vi "PWRMeasureCurrent.vi"(0 "PWR In":refnum<visa-resource-name>, 2 "Channel":string="1", 5 "error in (no error)":errorcluster {"code" format="%.0x"}, 6 "PWRID":u8) -> (14 "PWR Out":refnum<visa-resource-name>, 16 "Current Level (A)":dbl, 19 "error out":errorcluster)   [LabVIEW 2015]
uses:
  <instrlib>/Agilent N6700 Series/Agilent N6700 Series.lvlib
  <instrlib>/Agilent N87XX Series/Agilent N87XX Series.lvlib
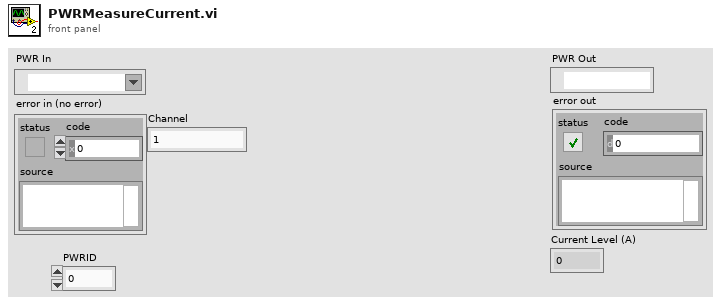
[diagram p1: front panel]
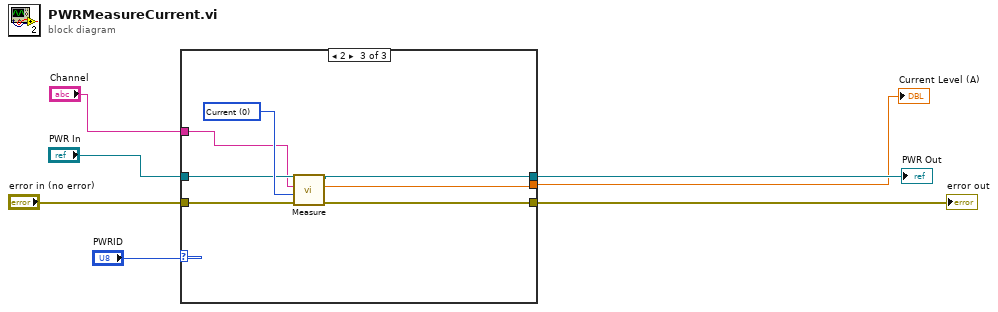
[diagram p0: block diagram]
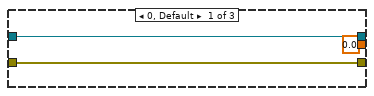
[diagram p2: hidden frame]
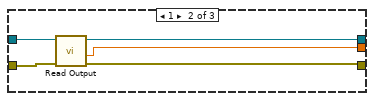
[diagram p3: hidden frame]
diagram:
  n1 = case shown="2" "PWRID" {
    tunnel: "PWR In" -> [w10 w15 w21]
    tunnel: "error in (no error)" -> [w9 w14 w20]
    tunnel: [w10 w13 w18] -> w5
    tunnel: [w9 w12 w17] -> w4
    tunnel: "Channel" -> [_ _ w19]
    tunnel: [0.0 ("Measurement") w11 w16] -> w1
    frame 0, Default {
    }
    frame 1 {
      n2 = call <instrlib>:"Read Output.vi"("error in (no error)"=w14, "VISA resource name"=w15) -> ("error out"=w12:errorcluster, "Actual Current Level (A)"=w11:dbl, "VISA resource name out"=w13:refnum<visa-resource-name>)  [unwired: 6 in, 1 out]
    }
    frame 2 {
      w22 = 0 items=["Current", "Voltage", "Power"] ("Measurement Type (1: Voltage)")
      n3 = call <instrlib>:"Measure.vi"("error in (no error)"=w20, "Measurement Type (1: Voltage)"=w22, "Channel Name (1)"=w19, "VISA resource name"=w21) -> ("error out"=w17:errorcluster, "Measurement"=w16:dbl, "VISA resource name out"=w18:refnum<visa-resource-name>)  [unwired: 5 in]
    }
  }
  "PWR Out" <- w5
  "error out" <- w4
  "Current Level (A)" <- w1
